vi "RoomReportDataToGraph3d.vi"(8 "error in (no error)":errorcluster, 9 "Bar References":refnum<vi>[](array[refnum]), 10 "Pie References":refnum<vi>[](array[refnum]), 11 "RoomReport":T2) -> (0 "error out":errorcluster, 1 "Bar Graphs":refnum<class "3D Plot Datatype.lvclass">[][](array[class]), 2 "Pie Graphs":refnum<class "3D Plot Datatype.lvclass">[][](array[class]))   [LabVIEW 2015]
uses:
  TypeDef/RoomReport.ctl
  <vilib>/Math Plots/3D Math Plots/3D Bar/3D Bar XCtrl/3D Bar.xctl
  <vilib>/Math Plots/3D Math Plots/3D Pie/3D Pie XCtrl/3D Pie.xctl
  TypeDef/RoomReportGraphs.ctl
  <vilib>/Math Plots/3D Math Plots/3D Plot/3D Plot Datatype/3D Plot Datatype.lvclass
  <vilib>/Math Plots/3D Math Plots/3D Pie/3D Pie Datatype/Public/Plot Helper (Vector).vi
  <vilib>/Math Plots/3D Math Plots/3D Bar/3D Bar Datatype/Public/Plot Helper (Matrix).vi
  <vilib>/Math Plots/3D Math Plots/3D Bar/3D Bar Datatype/3D Bar Datatype.lvclass
  <vilib>/Math Plots/3D Math Plots/3D Pie/3D Pie Datatype/3D Pie Datatype.lvclass
panel:
  out "NumNurseAlarmsPerRoom":i32[](array[numeric])
  out "NumDrAlarmsPerRoom":i32[](array[numeric])
  out "x+y":i32[](array[numeric])
  out "RoomGraphs":T1 {"NurseAvgFulfillTime(s)" scale=0.0..100.0; "DrAvgFulfillTime(s)" scale=0.0..200.0; "#NurseAlarms" scale=0.0..10.0; "#Patients" scale=0.0..10.0; "#DrAlarms" scale=0.0..10.0; "AvgStayPerRoom(s)" scale=0.0..10.0}
  out "Request With Alarm":refnum<class "3D Plot Datatype.lvclass">[](xcontrol)
  out "Number of Patients per Room":refnum<class "3D Plot Datatype.lvclass">[](xcontrol)
  out "Avg  Dr Complete Time":refnum<class "3D Plot Datatype.lvclass">[](xcontrol)
  out "Nurse Alarms":refnum<class "3D Plot Datatype.lvclass">[](xcontrol)
  out "Dr Alarms":refnum<class "3D Plot Datatype.lvclass">[](xcontrol)
  out "# Pattients Per Room":refnum<class "3D Plot Datatype.lvclass">[](xcontrol)
  out "Update":bool
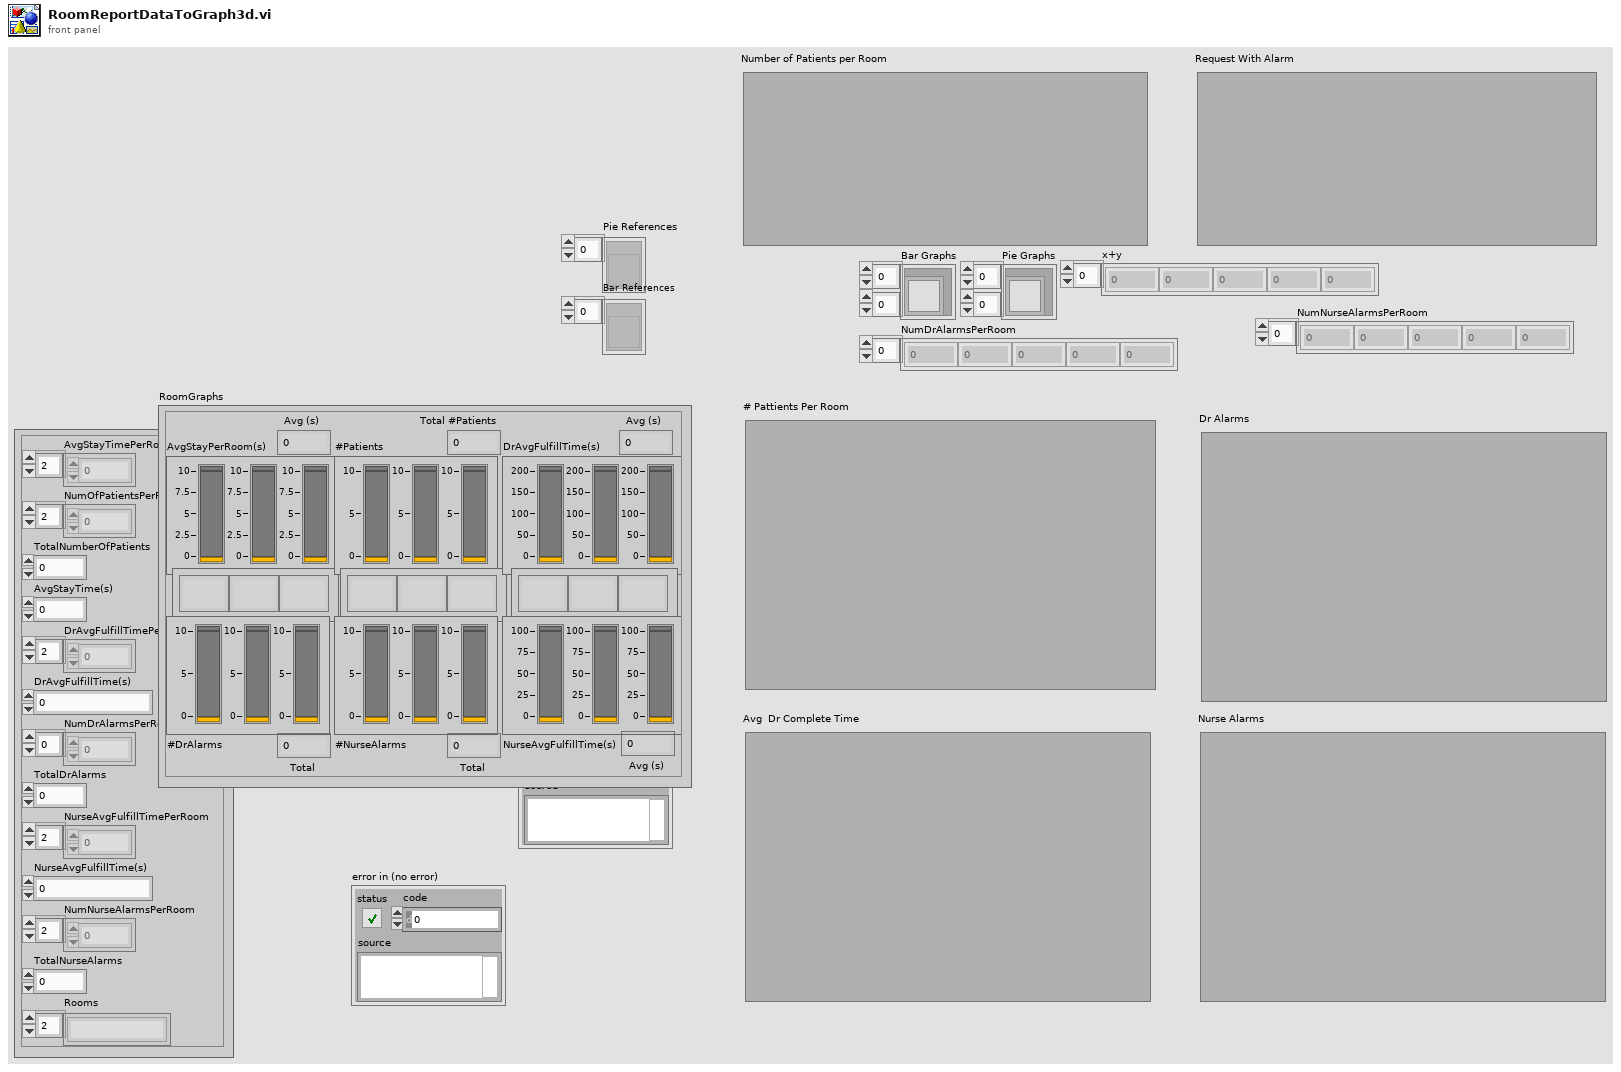
[diagram p1: front panel]
types:
  T1 = typedef "RoomReportGraphs.ctl" = cluster{"AvgStay (s)":dbl, "AvgStayPerRoom(s)":dbl[], "Total #Patients":i32, "#Patients":i32[], "TotalDrAvgFulfillTime(s)":dbl, "DrAvgFulfillTime(s)":dbl[], "#DrAlarms":i32[], "TotalDrAlarms":i32, "#NurseAlarms":i32[], "TotalNurseAlarms":i32, "NurseAvgFulfillTime(s)":dbl[], "TotalNurseAvgFulfillTime(s)":dbl, "RoomNumArr1":string[], "RoomNumArr2":string[], "RoomNumArr3":string[]}
  T2 = typedef "RoomReport.ctl" = cluster{"AvgStayTimePerRoom":dbl[], "NumOfPatientsPerRoom":i32[], "TotalNumberOfPatients":i32, "AvgStayTime(s)":dbl, "DrAvgFulfillTimePerRoom":dbl[], "DrAvgFulfillTime(s)":dbl, "NumDrAlarmsPerRoom":i32[], "TotalDrAlarms":i32, "NurseAvgFulfillTimePerRoom":dbl[], "NurseAvgFulfillTime(s)":dbl, "NumNurseAlarmsPerRoom":i32[], "TotalNurseAlarms":i32, "Rooms":string[]}
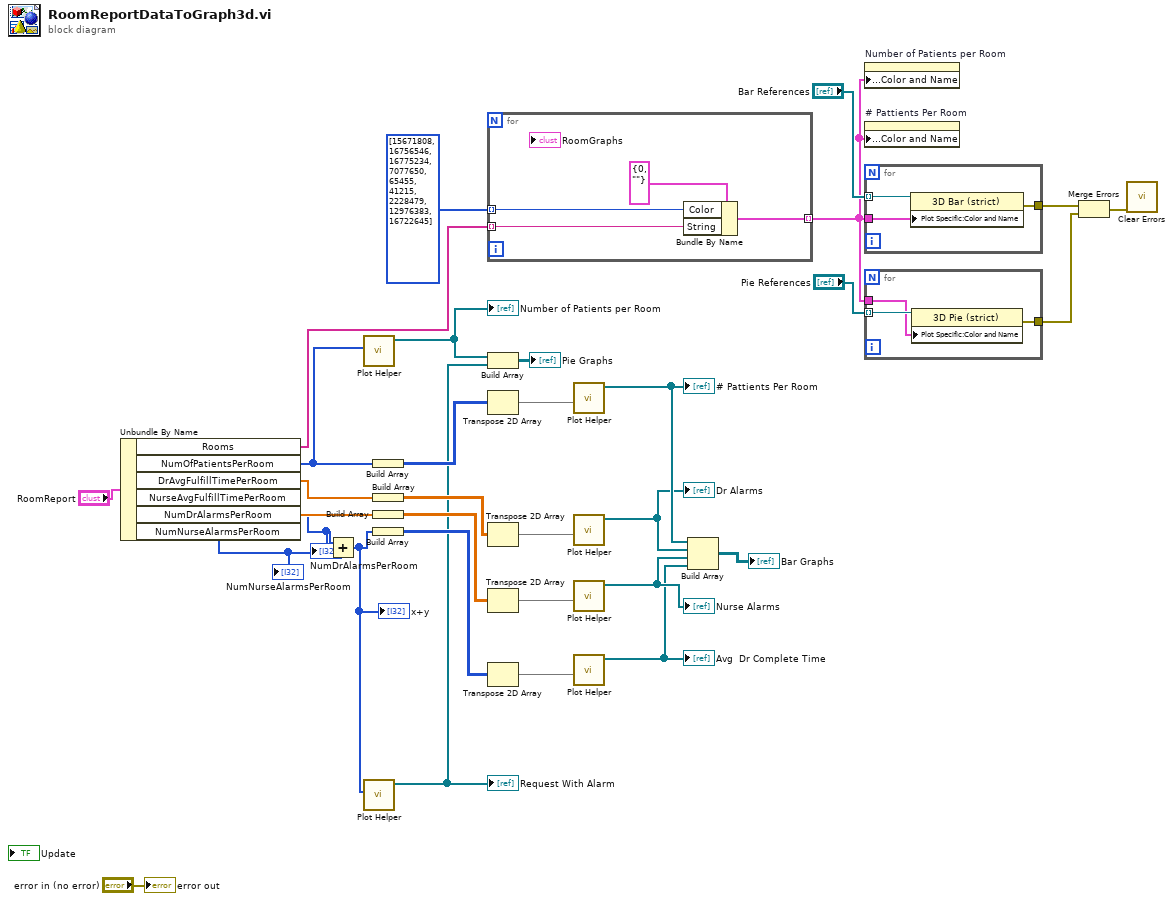
[diagram p0: block diagram]
diagram:
  n1 = Unbundle By Name("RoomReport") -> ("Rooms"=w16:string[], "NumOfPatientsPerRoom"=w12:i32[], "DrAvgFulfillTimePerRoom"=w15:dbl[], "NurseAvgFulfillTimePerRoom"=w14:dbl[], "NumDrAlarmsPerRoom"=w3:i32[], "NumNurseAlarmsPerRoom"=w2:i32[])
  "NumDrAlarmsPerRoom" <- w3
  "NumNurseAlarmsPerRoom" <- w2
  n2 = Add(x=w3, y=w2) -> (x+y=w1:i32[])
  "x+y" <- w1
  n3 = call-poly <vilib>:"Plot Helper.vi"("x vector"=w12) -> ("3D Plot lvclass Array out"=w9:refnum<class "3D Plot Datatype.lvclass">[])  [unwired: 2 in, 8 out]
  "Number of Patients per Room" <- w9
  n4 = call-poly <vilib>:"Plot Helper.vi"("x vector"=w1) -> ("3D Plot lvclass Array out"=w8:refnum<class "3D Plot Datatype.lvclass">[])  [unwired: 2 in, 8 out]
  "Request With Alarm" <- w8
  n5 = Build Array(w12) -> (w30:i32[][])
  n6 = Build Array(w15) -> (w29:dbl[][])
  n7 = Build Array(w14) -> (w26:dbl[][])
  n8 = Build Array(w1) -> (w13:i32[][])
  n9 = for {
    tunnel: [w35] -> w21 mode=indexing
    tunnel: u32[] [15671808, 16756546, 16775234, 7077650, 65455, 41215, 2228479, 12976383, 16722645] -> [w34] mode=indexing
    tunnel: w16 -> [w33] mode=indexing
    n10 = Bundle By Name(cluster=cluster{"Color":u32, "String":string} {"Color"=0, "String"=""} ("Color Pair"), "Color"=w34, "String"=w33) -> (w35:cluster{"Color":u32, "String":string})
  }
  n11 = Build Array(w9, w8) -> (→"Pie Graphs":refnum<class "3D Plot Datatype.lvclass">[][])
  n12 = Transpose 2D Array(2D array=w30) -> (transposed array=w24:i32[][])
  n13 = Transpose 2D Array(2D array=w29) -> (transposed array=w28:dbl[][])
  n14 = Transpose 2D Array(2D array=w26) -> (transposed array=w27:dbl[][])
  n15 = Transpose 2D Array(2D array=w13) -> (transposed array=w25:i32[][])
  n16 = call-poly <vilib>:"Plot Helper.vi"("z matrix"=w24) -> ("3D Plot lvclass Array out"=w11:refnum<class "3D Plot Datatype.lvclass">[])  [unwired: 2 in, 8 out]
  "# Pattients Per Room" <- w11
  n17 = call-poly <vilib>:"Plot Helper.vi"("z matrix"=w28) -> ("3D Plot lvclass Array out"=w6:refnum<class "3D Plot Datatype.lvclass">[])  [unwired: 2 in, 8 out]
  "Dr Alarms" <- w6
  n18 = call-poly <vilib>:"Plot Helper.vi"("z matrix"=w27) -> ("3D Plot lvclass Array out"=w5:refnum<class "3D Plot Datatype.lvclass">[])  [unwired: 2 in, 8 out]
  "Nurse Alarms" <- w5
  n19 = call-poly <vilib>:"Plot Helper.vi"("z matrix"=w25) -> ("3D Plot lvclass Array out"=w4:refnum<class "3D Plot Datatype.lvclass">[])  [unwired: 2 in, 8 out]
  "Avg  Dr Complete Time" <- w4
  n20 = Build Array(w11, w6, w5, w4) -> (→"Bar Graphs":refnum<class "3D Plot Datatype.lvclass">[][])
  n21 = property on="Number of Patients per Room" class="3D Pie (strict)"("Plot Specific:Color and Name"=w21) -> ()  [unwired: 2 in, 2 out]
  n22 = property on="# Pattients Per Room" class="3D Bar (strict)"("Plot Specific:Color and Name"=w21) -> ()  [unwired: 2 in, 2 out]
  n23 = for {
    tunnel: "Bar References" -> [w39] mode=indexing
    tunnel: w21 -> [w38]
    tunnel: [w37] -> w20
    n24 = property class="3D Bar (strict)"(reference=w39, "Plot Specific:Color and Name"=w38) -> (error out=w37:errorcluster)  [unwired: 1 in, 1 out]
  }
  n25 = for {
    tunnel: "Pie References" -> [w42] mode=indexing
    tunnel: w21 -> [w41]
    tunnel: [w40] -> w19
    n26 = property class="3D Pie (strict)"(reference=w42, "Plot Specific:Color and Name"=w41) -> (error out=w40:errorcluster)  [unwired: 1 in, 1 out]
  }
  n27 = Merge Errors(w20, w19) -> (w18:errorcluster)
  n28 = call <vilib>:"Clear Errors.vi"("error in (no error)"=w18) -> ()  [unwired: 5 in, 2 out]
  "error out" <- "error in (no error)"
